vi "make window modal until timeout.vi"(11 "timeout (ms)":i32=20000) -> ()   [LabVIEW 2017]
doc: "SciScan 1.2 160622"
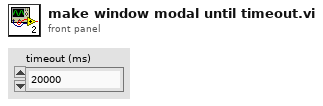
[diagram p1: front panel]
types:
  T1 = enum32{"Invalid", "Default", "Floating", "Floating/Auto-Hide", "Modal"}
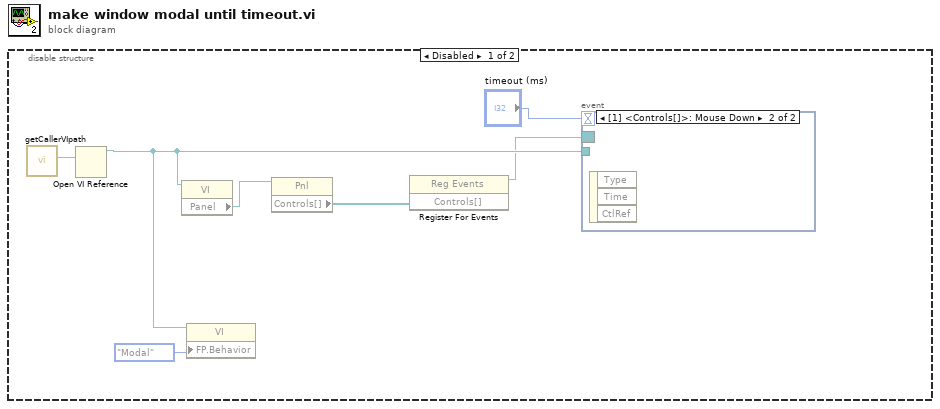
[diagram p0: block diagram]
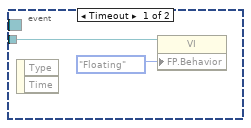
[diagram p2: hidden frame]
diagram:
  n1 = disable-structure shown="Disabled" {
    frame Disabled {
      n2 = call "getCallerVIpath.vi"() -> ("calling VI's absolute path"=w6:path)  [unwired: 10 in, 1 out]
      n3 = Open VI Reference(vi path=w6) -> (vi reference=w4:refnum<vi>)  [unwired: 5 in, 1 out]
      n4 = property class="VI"(reference=w4) -> ("Panel"=w3:refnum<vi>)  [unwired: 1 in, 2 out]
      n5 = property class="VI"(reference=w4, "FP.Behavior"=T1."Modal" ("Front Panel Window:Behavior")) -> ()  [unwired: 1 in, 2 out]
      n6 = property class="Pnl"(reference=w3) -> ("Controls[]"=w2:refnum<vi>[])  [unwired: 1 in, 2 out]
      n7 = register-events(w2) -> (reference out=w1:refnum<event-registration>)  [unwired: 2 in, 1 out]
      n8 = event shown="[1] <Controls[]>: Mouse Down" {
        selector: w1 -> [_ _]
        dyn-events: _ -> [_ _]
        timeout: "timeout (ms)" -> [_ _]
        tunnel: w4 -> [w9 _]
        event Timeout {
          n9 = event-data() -> ()  [unwired: 1 in, 2 out]
          n10 = property class="VI"(reference=w9, "FP.Behavior"=T1."Floating" ("Front Panel Window:Behavior")) -> ()  [unwired: 1 in, 2 out]
        }
        event Mouse Down {
          n11 = event-data() -> ()  [unwired: 1 in, 3 out]
        }
      }
    }
    frame Enabled {
    }
  }
